vi "_PC_Toolbar_Model_SetLayoutFix.vi"(1 "Tag":string, 2 "ToolBar_Panel_Ref":refnum<vi>) -> (0 "TotalWidth":i32)   [LabVIEW 2018]
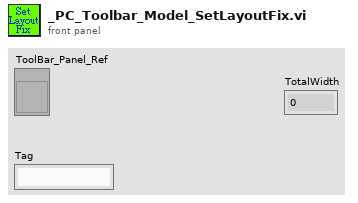
[diagram p1: front panel]
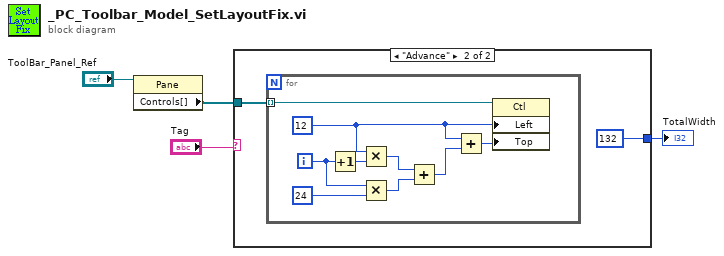
[diagram p0: block diagram]
diagram:
  n1 = property class="Pane"(reference="ToolBar_Panel_Ref") -> ("Controls[]"=w3:refnum<vi>[])  [unwired: 1 in, 2 out]
  n2 = case shown="\"Advance\"" "Tag" {
    tunnel: w3 -> [_ w6]
    tunnel: [_ 132] -> w2
    frame "False", Default {
    }
    frame "Advance" {
      n3 = for {
        tunnel: w6 -> [w10] mode=indexing
        i -> [w12]
        w8 = 12
        n4 = Increment(x=w12) -> (x+1=w15:i32)
        n5 = Multiply(x=w8, y=w15) -> (x*y=w14:i32)
        n6 = Multiply(x=w12, y=24) -> (x*y=w11:i32)
        n7 = Add(x=w14, y=w11) -> (x+y=w9:i32)
        n8 = Add(x=w8, y=w9) -> (x+y=w7:i32)
        n9 = property class="Ctl"(reference=w10, "Left"=w8, "Top"=w7) -> ()  [unwired: 1 in, 2 out]
      }
    }
  }
  "TotalWidth" <- w2
